vi "Set standard setup.vi"(8 "error in (no error)":errorcluster, 11 "CCD in":refnum<class "CCD.lvclass">) -> (0 "error out":errorcluster, 3 "CCD out":refnum<class "CCD.lvclass">)   [LabVIEW 2018, in "CCD.lvclass"]
uses:
  CCD.lvclass
  <userlib>/atmcd32d.llb/AcquisitionMode_mode typedef.ctl
  <userlib>/atmcd32d.llb/TriggerMode_mode typedef.ctl
  <userlib>/atmcd32d.llb/HSSpeed_type typedef.ctl
  <userlib>/atmcd32d.llb/Shutter_type typedef.ctl
  <userlib>/atmcd32d.llb/Shutter_mode typedef.ctl
  <userlib>/atmcd32d.llb/ReadMode_mode typedef.ctl
  CCD.lvclass/CCD.ctl
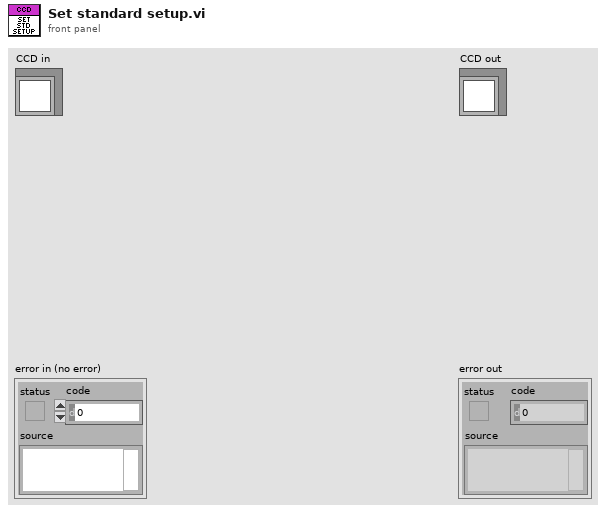
[diagram p1: front panel]
types:
  T1 = typedef "ReadMode_mode typedef.ctl" = enum16{"Full Vertical Binning", "Multi-Track", "Random-Track", "Single-Track", "Image"}
  T2 = typedef "Shutter_mode typedef.ctl" = enum16{"Auto", "Open", "Close", "N/A (3)", "Open FVB Series", "Open Any Series"}
  T3 = typedef "Shutter_type typedef.ctl" = enum16{"TTL Low", "TTL High"}
  T4 = typedef "HSSpeed_type typedef.ctl" = enum16{"EM Amp", "Conventional Amp"}
  T5 = typedef "TriggerMode_mode typedef.ctl" = enum16{"Internal", "External", "N/A (2)", "N/A (3)", "N/A (4)", "N/A (5)", "External Start", "External Exposure (Bulb)", "N/A (8)", "External FVB EM", "Software", "N/A (11)", "External Charge Shifting"}
  T6 = typedef "AcquisitionMode_mode typedef.ctl" = enum16{"Reserved (0)", "Single Scan", "Accumulate", "Kinetics", "Fast Kinetics", "Run Till Abort", "Reserved (6)", "Reserved (7)", "Reserved (8)", "Time Delayed Integration"}
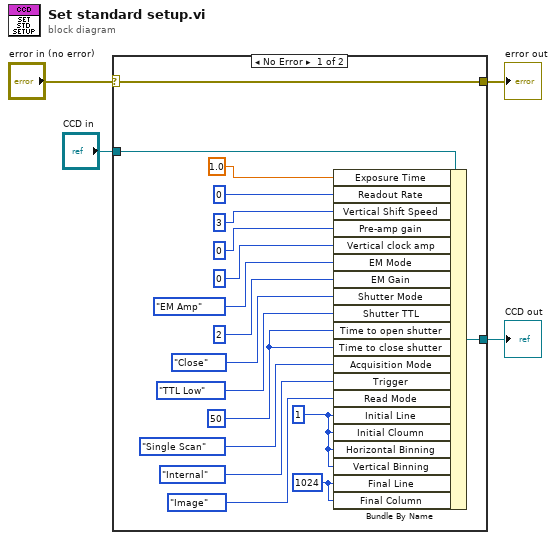
[diagram p0: block diagram]
diagram:
  n1 = case shown="No Error" "error in (no error)" {
    selector: "error in (no error)" -> [w22 w24]
    tunnel: [w22 w24] -> w2
    tunnel: [w20 w23] -> w1
    tunnel: "CCD in" -> [w21 w23]
    frame No Error {
      w5 = u16 1024 ("Initial Line")
      w6 = u16 1 ("Initial Line")
      w10 = u16 50 ("Time to open shutter")
      n2 = Bundle By Name(cluster=w21, "Exposure Time"=1.0, "Readout Rate"=u8 0, "Vertical Shift Speed"=u8 3, "Pre-amp gain"=u8 0, "Vertical clock amp"=u8 0, "EM Mode"=HSSpeed_type_typedef."EM Amp" ("type"), "EM Gain"=u16 2, "Shutter Mode"=Shutter_mode_typedef."Close" ("mode"), "Shutter TTL"=Shutter_type_typedef."TTL Low" ("type"), "Time to open shutter"=w10, "Time to close shutter"=w10, "Acquisition Mode"=AcquisitionMode_mode_typedef."Single Scan" ("mode"), "Trigger"=TriggerMode_mode_typedef."Internal" ("mode"), "Read Mode"=ReadMode_mode_typedef."Image" ("mode"), "Initial Line"=w6, "Initial Cloumn"=w6, "Horizontal Binning"=w6, "Vertical Binning"=w6, "Final Line"=w5, "Final Column"=w5) -> (w20:refnum<class "CCD.lvclass">)
    }
    frame Error {
    }
  }
  "error out" <- w2
  "CCD out" <- w1
